vi "LinDaten speichern und laden.vi"(6 "Aktion":enum16{"speichern", "laden"}(ring), 8 "error in (no error)":errorcluster caption="Fehler (Eingang, kein Fehler)", 9 "test Polynom":bool, 10 "Analysator":T2, 11 "selected path":path caption="Ausgewählter Pfad") -> (0 "error out":errorcluster caption="Fehler (Ausgang)", 1 "Daten zum Speichern":string[](array[string]), 2 "LIN Protokoll Daten":T4 {"zusätzliche Zeitdauer Erster Punkt" format="%#_5g"; "Lin Modus" items=["Cal Gas to PNS", "Cal Gas to Samplepoint", "Measure"]; "Gas Ablaufdatum" format="%<%d.%m.%Y>T"; "HovaCAL Flow AutoLin"."HovaCAL Flow Input Cluster" format="%.2f"; "Gasflasche" items=["----"=10000, "IAG MG"=0, "IAG NH3 3000"=1, "IAG NH3 2000"=2, "IAG NH3 200"=3]; "Conditions:" items=["field", "laboratory"]; "Kalibrierauswahl" items=["Inaktiv", "Aktiv"]; "Anzahl Stufen" format="%#_5g"; "Zeitdauer Stufe" format="%#_5g"; "Verdünnungsgas" items=["N2", "O2"]; "Komponentenauswahl"."Konzentration" format="%#.6f"; "Gasnummer:" min=1 max=5; "Prüfgas Konzentration" format="%#.6f"; "Polynomkoeff." format="%#_18f"}, 3 "MessDaten Array":string[][][](array[string]), 4 "Ident Cluster":T18, 5 "Setup Daten-Cluster":T3, 7 "Settings Cluster":T1)   [LabVIEW 2020, in "Linearisierung v2.lvlib"]
uses:
  Linearisierung v2.lvlib
  SpanEinstellungen/LIN Loading Errors.ctl
  Lin-Polynom Daten.ctl
  KomponentenArray.ctl
  Visualisierungs Elemente/Auswahlfeld.ctl
  Visualisierungs Elemente/Zahlen-Eingabefeld.ctl
  EPA Optionsfeld.ctl
  Gasteiler/HovaCal/AutoLin Hovacal.ctl
  Kalibrieroption.ctl
  EPA1065-307/Condition.ctl
  Seiten/System Einstellungen V2/Konfig Gasflasche.ctl
  Seiten/System Einstellungen V2/Gasflasche Auswahl.ctl
  Gasteiler/HovaCAL_Interface/Controls/Flow Einstellung.ctl
  Gasteiler/HovaCAL_Interface/Controls/Pump state.ctl
  Seiten/CalGas Aufschaltung/Lin Modus.ctl
  SpanEinstellungen/LIN Loading Setup Data.ctl
  Seiten/System Einstellungen V2/Analysatoren.ctl
  Aktion Lin Daten aufarbeiten.ctl
  Seiten/FT-IR/FGV FT-IR Gasliste Aktionen.ctl
  Seiten/FT-IR/FGV FT-IR Aktionen.ctl
  Seiten/System Einstellungen V2/Aktioen FGV System Konstanten.ctl
  Seiten/System Einstellungen V2/Aktion FGV SystemEinstellungenV2.ctl
  Gasteiler/Aktionen FGV Gasteiler Daten.ctl
  PDF_Interface/PDF Protokoll Standard Kopf Gasflasche Auswahl.ctl
  SpanEinstellungen/Aktion FGV SpanEinstellungen.ctl
  Seiten/FT-IR/Span/Aktion FGV Span.ctl
  <vilib>/Utility/file.llb/Read Delimited Spreadsheet (string).vi
  Seiten/FT-IR/FT-IR.lvlib
  Seiten/System Einstellungen V2/System Einstellungen V2.lvlib
  Gasteiler/Gasteiler.lvlib
  PDF_Interface/PDF Interface.lvlib
  SpanEinstellungen/SpanEinstellungen.lvlib
  Seiten/FT-IR/Span/Spanfaktor.lvlib
  Protokoll/Protokoll.lvlib
  Gasteiler/HovaCal/HovaCal.lvlib
  EPA1065-307/Linearity verification 1065-307.lvlib
  Gasteiler/HovaCAL_Interface/Controls/Controls.lvlib
  Seiten/CalGas Aufschaltung/CalGas Aufschaltung.lvlib
panel:
  # "%"
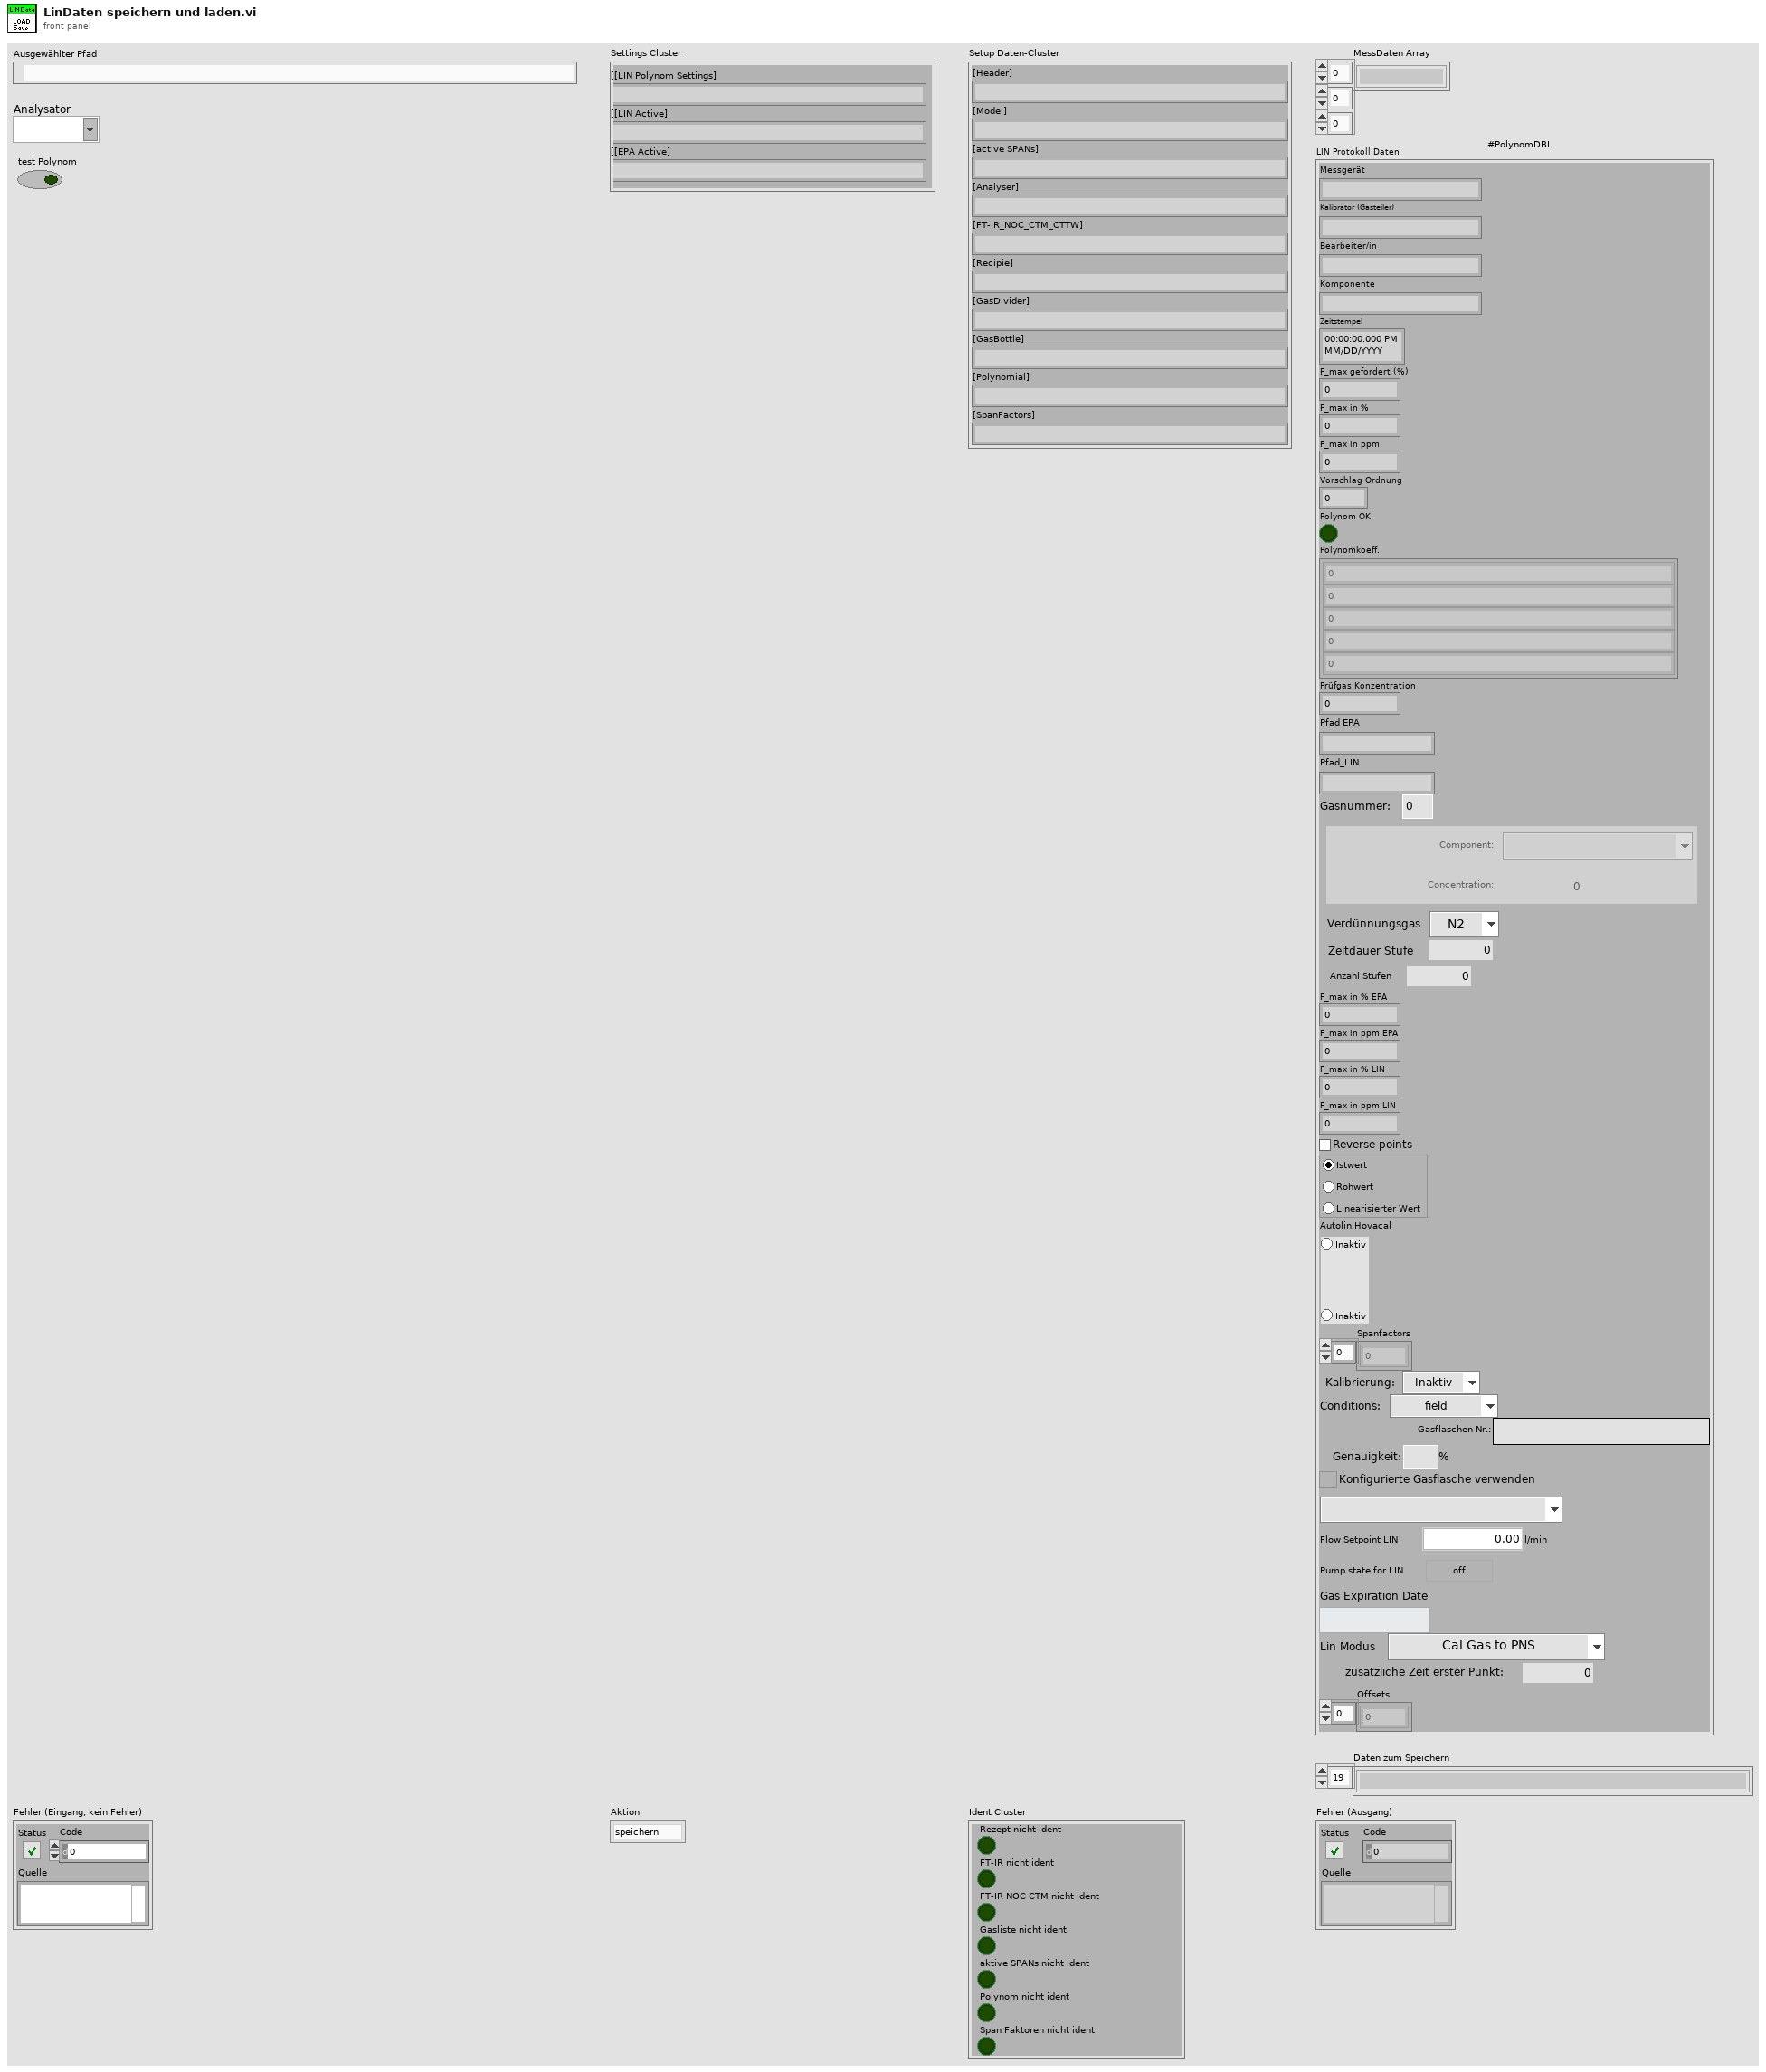
[diagram p1: front panel]
types:
  T1 = cluster{"[[LIN Polynom Settings]":string, "[[LIN Active]":string, "[[EPA Active]":string}
  T2 = typedef "System Einstellungen V2.lvlib/Analysatoren.ctl" = string
  T3 = typedef "Linearisierung v2.lvlib/SpanEinstellungen.lvlib/LIN Loading Setup Data.ctl" = cluster{"[Header]":string, "[Model]":string, "[active SPANs]":string, "[Analyser]":string, "[FT-IR_NOC_CTM_CTTW]":string, "[Recipie]":string, "[GasDivider]":string, "[GasBottle]":string, "[Polynomial]":string, "[SpanFactors]":string}
  T4 = typedef "Linearisierung v2.lvlib/Lin-Polynom Daten.ctl" = cluster{"Messgerät":string, "Kalibrator (Gasteiler)":string, "Bearbeiter/in":string, "Komponente":string, "Zeitstempel":timestamp, "F_max gefordert (%)":sgl, "F_max in %":sgl, "F_max in ppm":sgl, "Vorschlag Ordnung":i32, "Polynom OK":bool, "Polynomkoeff.":dbl[], "Prüfgas Konzentration":dbl, "Pfad EPA":string, "Pfad_LIN":string, "Gasnummer:":u8, "Komponentenauswahl":T5, "Verdünnungsgas":T7, "Zeitdauer Stufe":T8, "Anzahl Stufen":T8, "F_max in % EPA":sgl, "F_max in ppm EPA":sgl, "F_max in % LIN":sgl, "F_max in ppm LIN":sgl, "Punkte umkehren":bool, "EPA Optionsfeld":T9, "Autolin Hovacal":T10, "Spanfactors":sgl[], "Kalibrierauswahl":T11, "Conditions:":T12, "Gasflaschen Nr.:":string, "Bottle Accuracy":dbl, "Konfig Gasflasche":T13, "Gasflasche":T14, "HovaCAL Flow AutoLin":T15, "MFC Output":T16, "Gas Ablaufdatum":timestamp, "Lin Modus":T17, "zusätzliche Zeitdauer Erster Punkt":sgl, "Offsets":sgl[]}
  T5 = typedef "Linearisierung v2.lvlib/KomponentenArray.ctl" = cluster{"Komponente:":T6, "Konzentration":dbl}[]
  T6 = typedef "Auswahlfeld.ctl" = u16
  T7 = typedef "Linearisierung v2.lvlib/Gasteiler.lvlib/Prüfgas in.ctl" = u16
  T8 = typedef "Zahlen-Eingabefeld.ctl" = sgl
  T9 = typedef "Linearisierung v2.lvlib/EPA Optionsfeld.ctl" = enum32{"Istwert", "Rohwert", "Linearisierter Wert"}
  T10 = typedef "Linearisierung v2.lvlib/Gasteiler.lvlib/HovaCal.lvlib/AutoLin Hovacal.ctl" = enum32{"Keine Auswahl", "Optionsauswahl 1", "Optionsauswahl 2"}
  T11 = typedef "Linearisierung v2.lvlib/Kalibrieroption.ctl" = u16
  T12 = typedef "Linearisierung v2.lvlib/Linearity verification 1065-307.lvlib/Condition.ctl" = u16
  T13 = typedef "System Einstellungen V2.lvlib/Konfig Gasflasche.ctl" = bool
  T14 = typedef "System Einstellungen V2.lvlib/Gasflasche Auswahl.ctl" = u16
  T15 = typedef "Linearisierung v2.lvlib/Gasteiler.lvlib/HovaCAL_Interface.lvlib/Controls.lvlib/Flow Einstellung.ctl" = cluster{"HovaCAL Flow Input Cluster":dbl}
  T16 = typedef "Linearisierung v2.lvlib/Gasteiler.lvlib/HovaCAL_Interface.lvlib/Controls.lvlib/Pump state.ctl" = cluster{"Run":bool}
  T17 = typedef "CalGas Aufschaltung.lvlib/Lin Modus.ctl" = u16
  T18 = typedef "Linearisierung v2.lvlib/SpanEinstellungen.lvlib/LIN Loading Errors.ctl" = cluster{"Rezept nicht ident":bool, "FT-IR nicht ident":bool, "FT-IR NOC CTM nicht ident":bool, "Gasliste nicht ident":bool, "aktive SPANs nicht ident":bool, "Polynom nicht ident":bool, "Span Faktoren nicht ident":bool}
  T19 = typedef "Linearisierung v2.lvlib/Protokoll.lvlib/Aktion LIN Polynom Ordnung je Komponente für Protokoll.ctl" = enum16{"lesen", "schreiben", "init", "schreiben viewonly", "init initial"}
  T20 = typedef "Linearisierung v2.lvlib/SpanEinstellungen.lvlib/Aktion FGV SpanEinstellungen.ctl" = enum16{"lesen", "schreiben", "laden", "speichern", "RegisterRef", "automatisch", "init", "PDF Params", "Punkte umkehren"}
  T21 = typedef "PDF Interface.lvlib/PDF Protokoll Standard Kopf Gasflasche Auswahl.ctl" = cluster{"Gasflaschen Name":string, "Gasflaschen Nummer":string, "Gasnummer Index":i32}
  T22 = typedef "Linearisierung v2.lvlib/Gasteiler.lvlib/Aktionen FGV Gasteiler Daten.ctl" = enum16{"lesen", "Gasteiler Daten", "Seriellen Param.", "MB-Endwert", "laden", "speichern", "Anforderung", "TCP", "Aufzeichnung Start"}
  T23 = typedef "System Einstellungen V2.lvlib/Aktion FGV SystemEinstellungenV2.ctl" = enum16{"lesen", "Analysatoren schreiben", "Analysator ändern", "Analysatoren löschen", "laden", "speichern", "Untertitel", "Analysatoren", "Neue Analysatoren", "Gasteiler schreiben", "Gasteiler ändern", "Gasteiler löschen", "Gasteiler", "Gasteiler exportieren", "Gasteiler importieren"}
  T24 = typedef "System Einstellungen V2.lvlib/Aktioen FGV System Konstanten.ctl" = enum16{"lesen", "laden", "speichern", "Sprache"}
  T25 = typedef "FT-IR.lvlib/FGV FT-IR Aktionen.ctl" = enum16{"lesen", "NOG setzen", "NOS setzen", "Initialisieren", "speichern", "ALLES setzen", "FT-IR Spektrum loggen", "Komm Stoppen", "Spektrum LogKonfig"}
  T26 = typedef "FT-IR.lvlib/FGV FT-IR Gasliste Aktionen.ctl" = enum16{"lesen", "Gasliste FT-IR", "Gasliste ausgelesen", "laden", "speichern", "löschen"}
  T27 = typedef "Linearisierung v2.lvlib/Aktion Lin Daten aufarbeiten.ctl" = enum16{"lesen", "Protkolldaten", "speichern", "laden", "EPA auswerten", "Tabelle schreiben", "Lin auswerten", "Tab init", "Stufentabelle", "EPA aktiviert", "Nachbehandlung laden", "Tabelle löschen", "Istwerte löschen", "Zeile löschen", "Zeile einfügen", "LIN aktiviert", "LIN/EPA aktiv laden", "EGAK Tab", "LIN übernehmen", "Tab init ohne Stufen"}
  T28 = typedef "FT-IR.lvlib/Spanfaktor.lvlib/Aktion FGV Span.ctl" = enum16{"lesen", "Span", "Seite aktiv", "Offset", "FGV aktualisiert", "Aktualisierung aufheben"}
  T29 = typedef "System Einstellungen V2.lvlib/Gasteiler.ctl" = cluster{"Gasteiler Name":string, "Gasteiler Type":string, "Gasteiler Seriennummer":string, "Gasteiler Letzte Wartung":timestamp}
  T30 = cluster{"GasteilerDefinitionsListe":T29[], "GasteilerDefinitionTextliste":string[][], "Gasteiler Strings And Values":cluster{"String":string, "Wert":string}[]}
  T31 = typedef "Linearisierung v2.lvlib/Gasteiler.lvlib/Gasteiler Daten.ctl" = cluster{"Gasteiler":T32, "Gasteiler Stufen":T33, "Gasteiler Type":T34, "Konfig Gasteiler":T35, "Gasteiler Span Eingänge":u16}
  T32 = typedef "String - Eingabefeld.ctl" = string
  T33 = typedef "Linearisierung v2.lvlib/Gasteiler.lvlib/Gasteiler Stufen.ctl" = u16
  T34 = typedef "Linearisierung v2.lvlib/GasteilerType.ctl" = u16
  T35 = typedef "System Einstellungen V2.lvlib/Gasteiler Auswahl.ctl" = u16
  T36 = typedef "Linearisierung v2.lvlib/AktivArray.ctl" = T37[]
  T37 = typedef "Linearisierung v2.lvlib/AktivButton.ctl" = bool
  T38 = typedef "String - Ausgabefeld.ctl" = string
  T39 = cluster{"Modell":string, "ProjektNummer":string, "Software Version":string, "Seriennummer":string}
  T40 = typedef "Linearisierung v2.lvlib/SpanEinstellungen.lvlib/SpanInletCluster.ctl" = cluster{"Span Inlet Active":T13, "Analysator":T2, "Konfig Gasflasche":T13, "Gasflasche":T14, "Gasflaschen Nr.:":string, "Ablaufdatum":timestamp, "Komponenten":T41, "Zeitdauer Stufen":sgl, "Max Fehler":sgl, "Anzahl Stufen":sgl, "Trägergas":T44, "zusätzliche Zeitdauer Erster Punkt":sgl}
  T41 = typedef "Linearisierung v2.lvlib/SpanEinstellungen.lvlib/Komponentencluster mit Formel.ctl" = cluster{"Komponente 1":T42, "Komponente 2":T42, "Komponente 3":T42, "Komponente 4":T42, "Komponente 5":T42}
  T42 = typedef "Linearisierung v2.lvlib/SpanEinstellungen.lvlib/Komponentenauswahl mit Formel.ctl" = cluster{"Komponente:":u16, "Summenformel":T32, "Konzentration IST":dbl, "Einheit":T43, "Genauigkeit":dbl}
  T43 = typedef "Linearisierung v2.lvlib/SpanEinstellungen.lvlib/Einheit.ctl" = enum16{"ppm", "%"}
  T44 = typedef "System Einstellungen V2.lvlib/Traegergas.ctl" = string
  T45 = typedef "Linearisierung v2.lvlib/Auswahl Polynom Ordnung.ctl" = enum16{"autom.", "raw", "actual", "1", "2", "3", "4"}
  T46 = cluster{"active SPAN Idx":i32, "active Component Index":i32}
  T47 = cluster{"spreadsheet string":string, "spreadsheet string":string, "spreadsheet string":string, "spreadsheet string":string, "spreadsheet string":string, "spreadsheet string":string, "spreadsheet string":string, "spreadsheet string":string, "spreadsheet string":string, "spreadsheet string":string}
  T48 = cluster{"spreadsheet string":string, "spreadsheet string":string, "spreadsheet string":string}
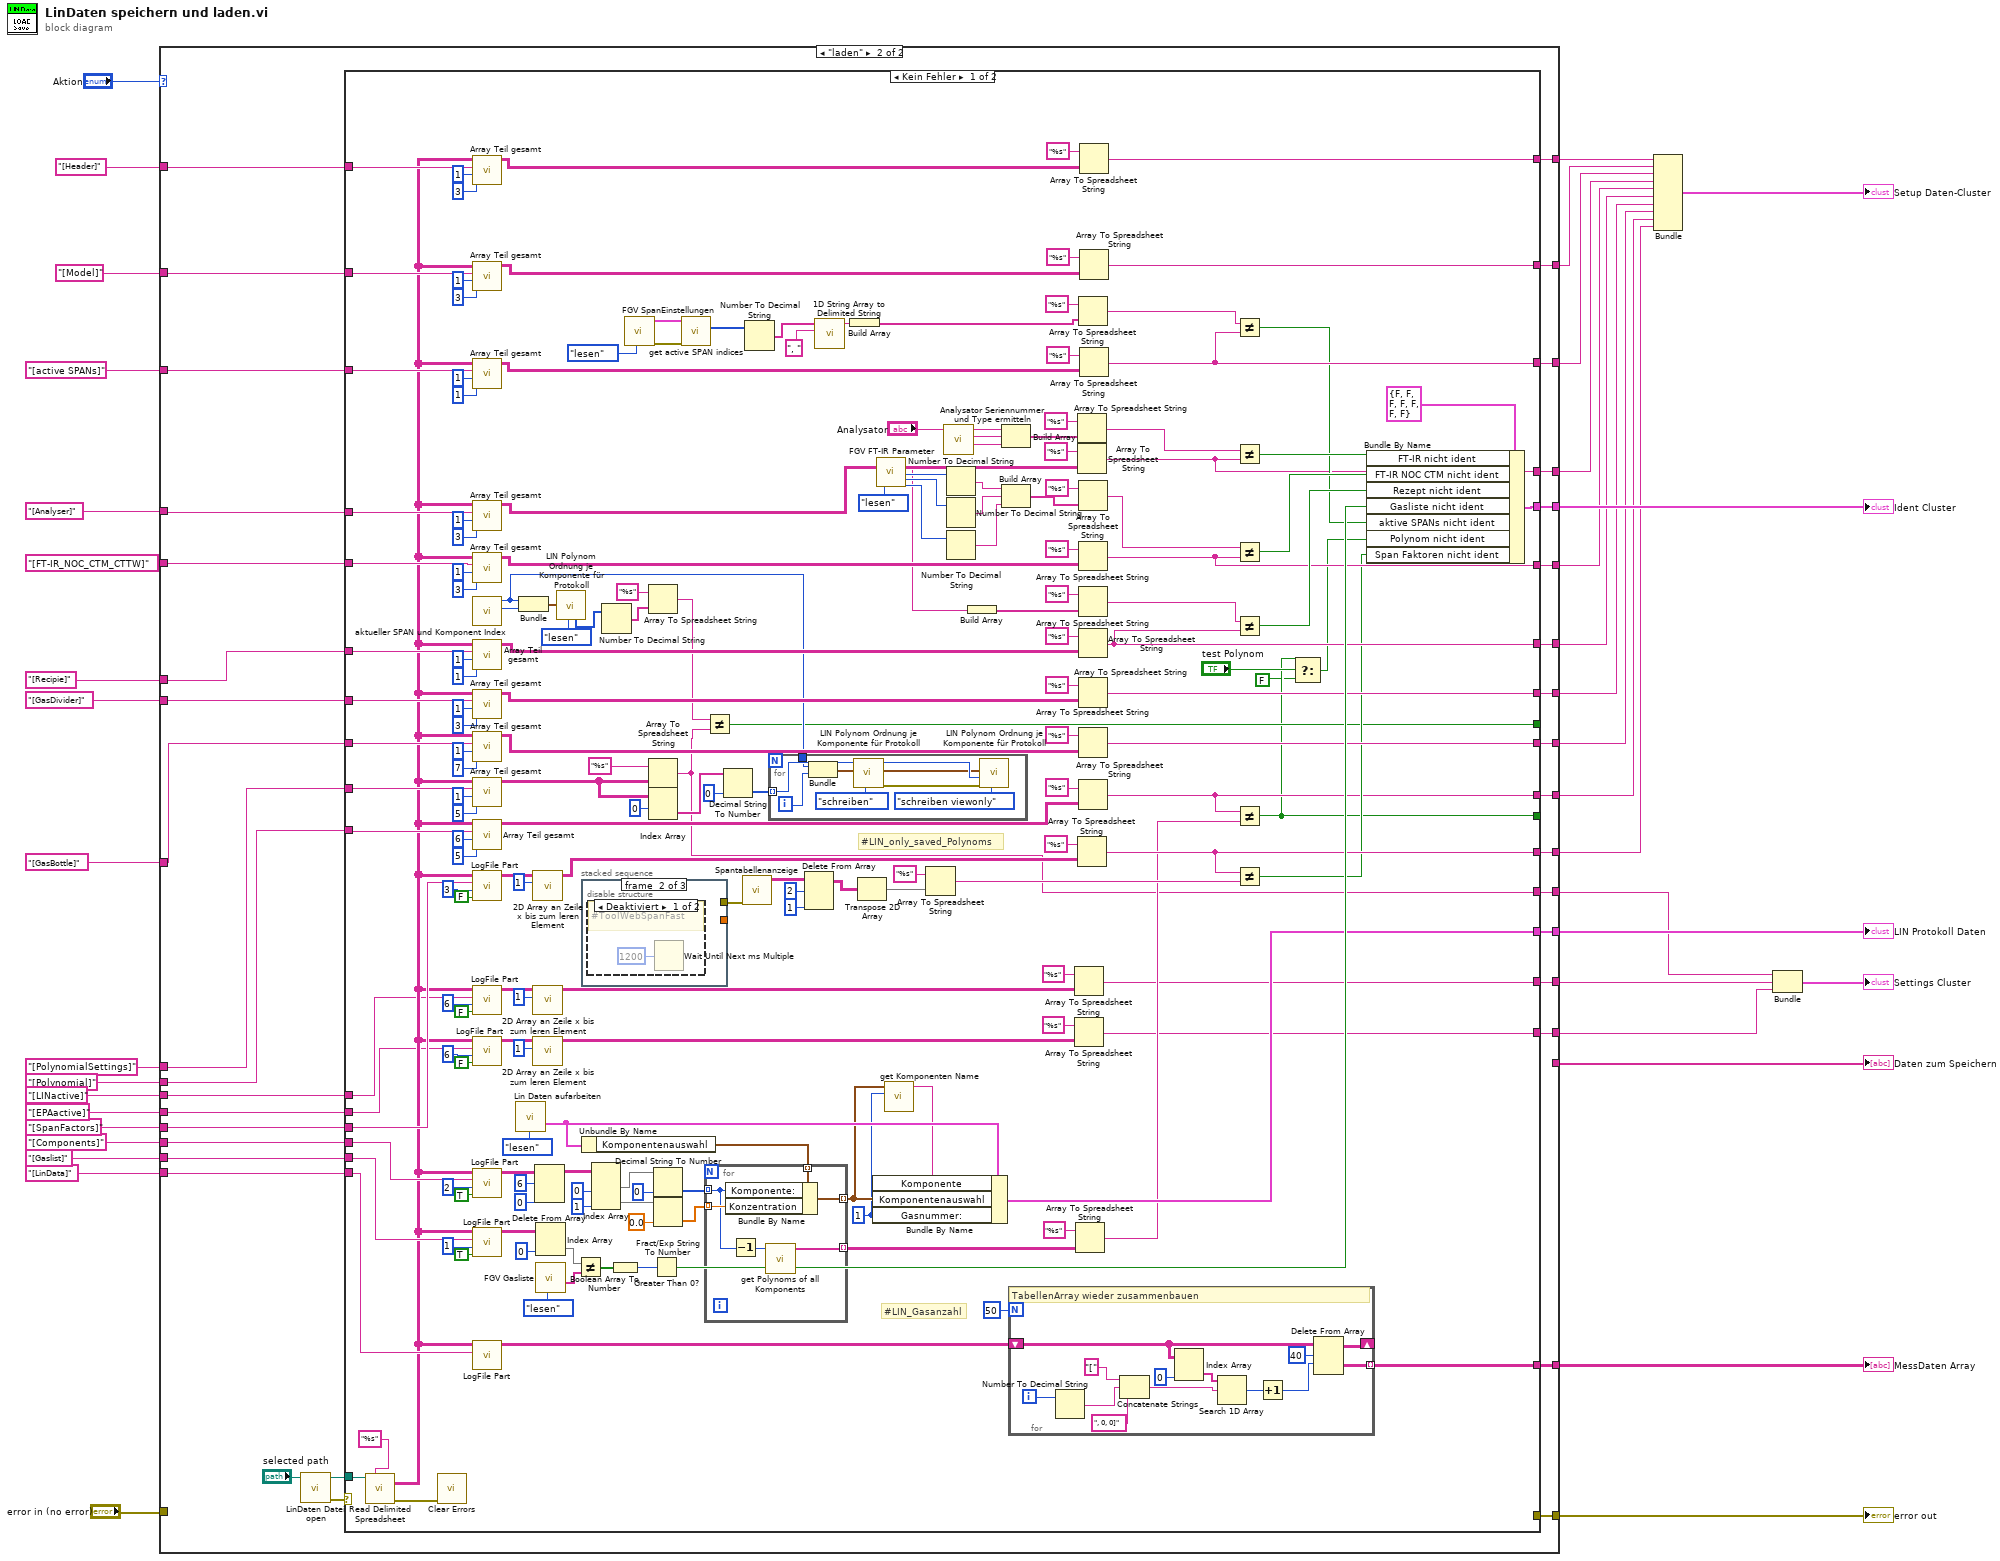
[diagram p0: block diagram]
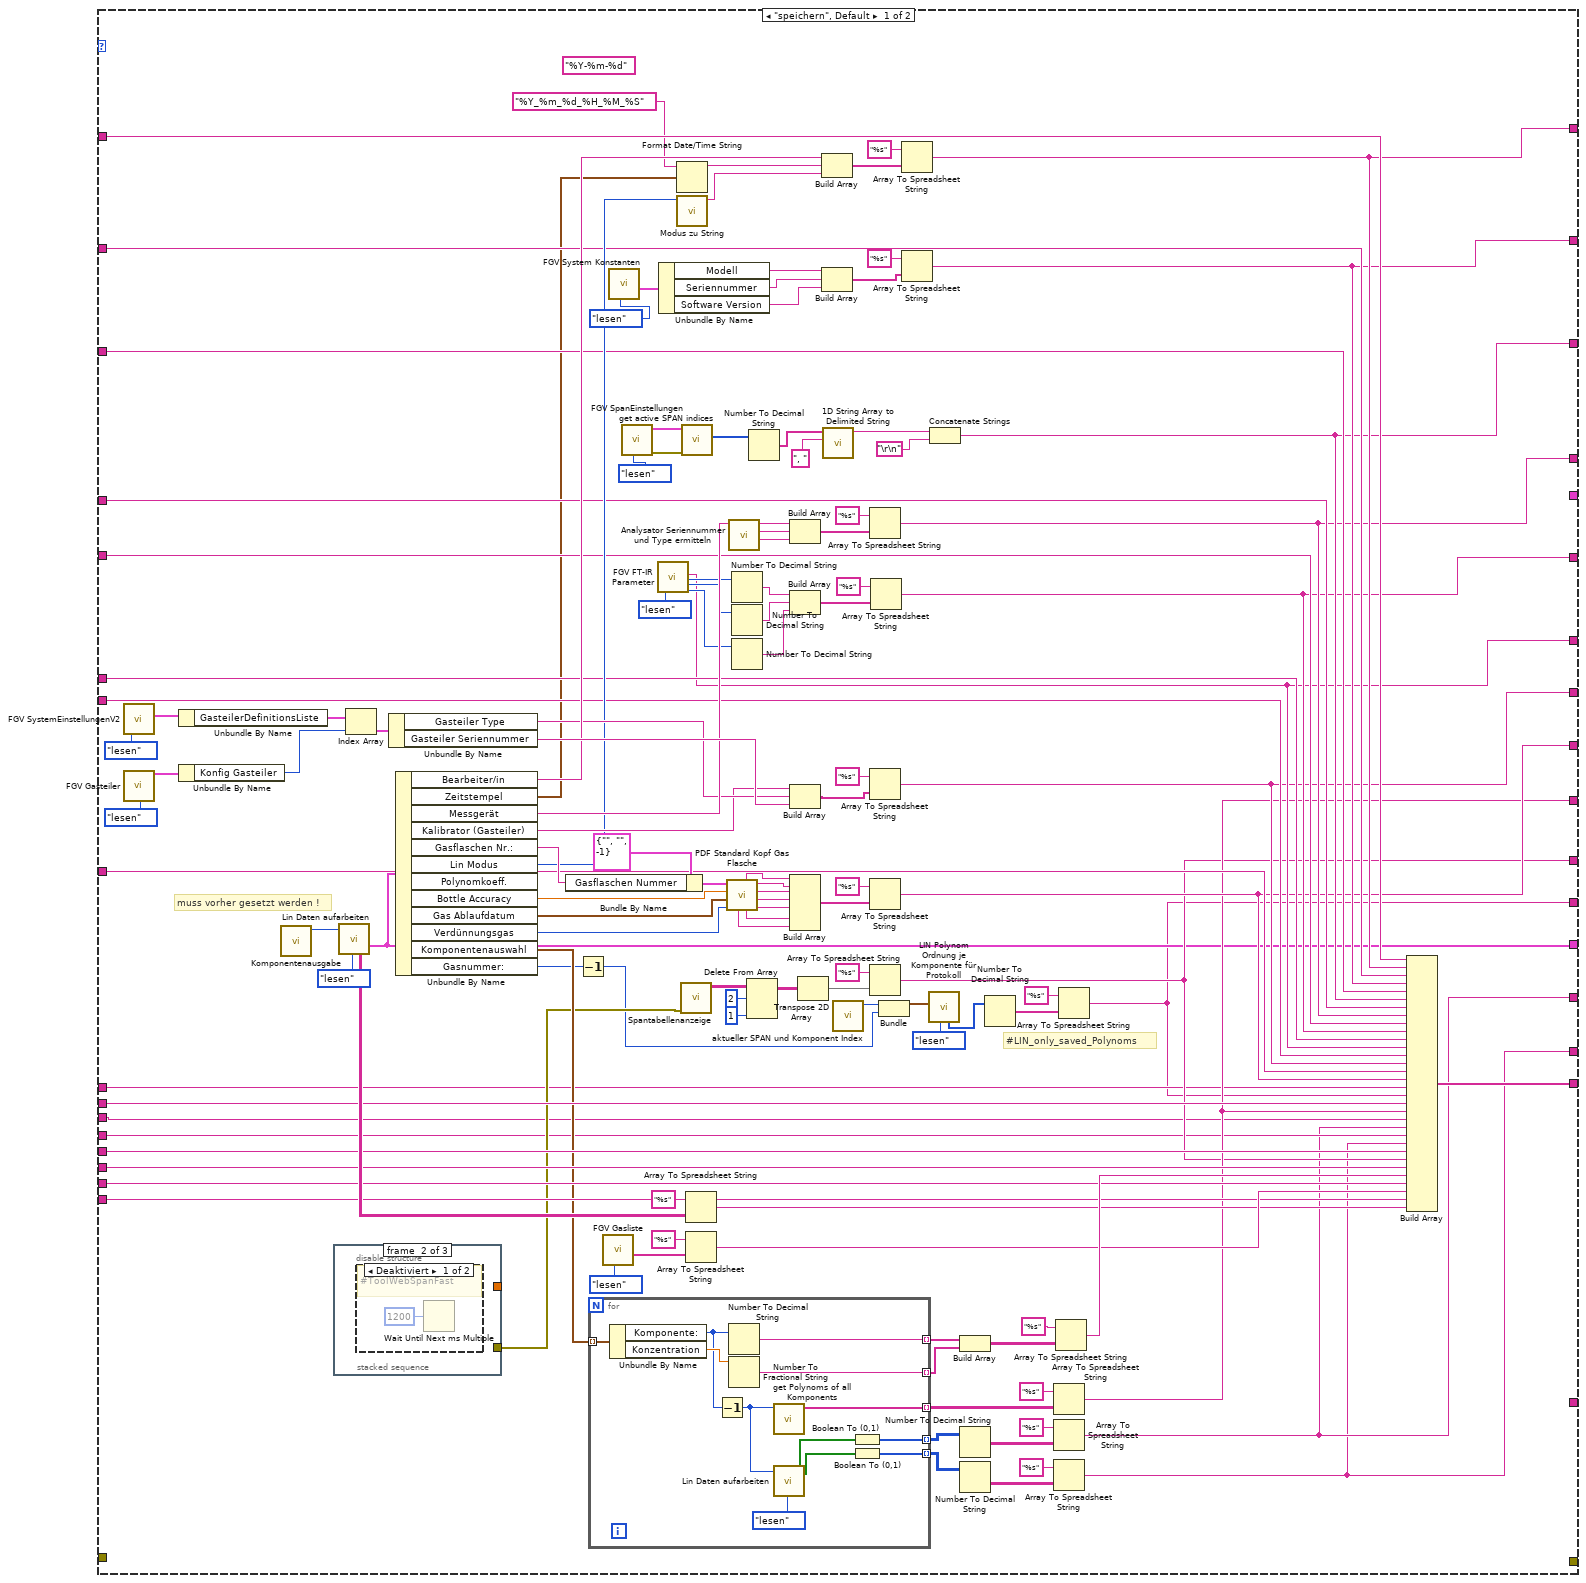
[diagram p2: hidden frame]
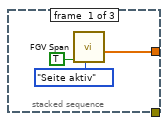
[diagram p3: hidden frame]
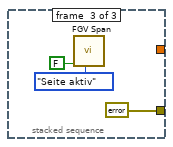
[diagram p5: hidden frame]
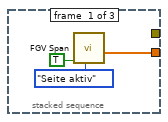
[diagram p6: hidden frame]
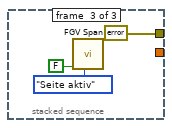
[diagram p8: hidden frame]
diagram:
  n1 = case shown="\"laden\"" "Aktion" {
    tunnel: [_ w225] -> w37
    tunnel: "[Header]" -> [w99 w213]
    tunnel: "[Model]" -> [w98 w214]
    tunnel: "[Analyser]" -> [w97 w215]
    tunnel: "[FT-IR_NOC_CTM_CTTW]" -> [w96 w216]
    tunnel: "[Recipie]" -> [w95 w217]
    tunnel: "[GasDivider]" -> [w94 w218]
    tunnel: "[GasBottle]" -> [w93 w219]
    tunnel: "[Polynomial]" -> [w92 w220]
    tunnel: "[SpanFactors]" -> [w91 w221]
    tunnel: "[Components]" -> [w90 w222]
    tunnel: "[Gaslist]" -> [w89 w224]
    tunnel: "[LinData]" -> [w88 w223]
    tunnel: [_ w212] -> w24
    tunnel: [w87 _] -> w23
    tunnel: "[active SPANs]" -> [w78 w210]
    tunnel: [w67 w209] -> w21
    tunnel: [_ w208] -> w20
    tunnel: [w77 w207] -> w19
    tunnel: [w76 w206] -> w18
    tunnel: [w75 w205] -> w17
    tunnel: [w71 w204] -> w13
    tunnel: [w70 w203] -> w12
    tunnel: [w69 w202] -> w11
    tunnel: [w68 w201] -> w10
    tunnel: [w74 w200] -> w16
    tunnel: [w73 w199] -> w15
    tunnel: [w72 w198] -> w14
    tunnel: "[PolynomialSettings]" -> [w58 w197]
    tunnel: "[LINactive]" -> [w43 w196]
    tunnel: "[EPAactive]" -> [w42 w195]
    tunnel: "error in (no error)" -> [_ _]
    tunnel: [w41 w194] -> w4
    tunnel: [w40 w193] -> w3
    tunnel: [w39 w192] -> w2
    frame "speichern", Default {
      (unwired) "%Y-%m-%d" ("Zeitformatierungs-String (%c)")
      # "muss vorher gesetzt werden !"
      # "#LIN_only_saved_Polynoms"
      n2 = call "FGV SystemEinstellungenV2.vi"("Aktion"=Aktion_FGV_SystemEinstellungenV2."lesen") -> ("Gasteiler"=w155:T30)  [unwired: 5 in, 5 out]
      n3 = call "FGV Gasteiler.vi"("Aktionen"=Aktionen_FGV_Gasteiler_Daten."lesen") -> ("Gasteiler Daten"=w153:T31)  [unwired: 11 in, 7 out]
      n4 = Unbundle By Name(w155) -> ("GasteilerDefinitionsListe"=w154:T29[])
      n5 = Unbundle By Name(w153) -> ("Konfig Gasteiler"=w151:T35)
      n6 = call "Komponentenausgabe.vi"() -> ("Gaskomponente"=w61:T6)  [unwired: 8 in, 3 out]
      n7 = stacked-sequence {
        tunnel: [w173 _ _] -> _
        tunnel: [_ _ errorcluster {"status"=FALSE, "code"=0, "source"=""} ("Fehlerkonstante")] -> w60
        frame #0 {
          n8 = call "FGV Span.vi"("Aktion"=Aktion_FGV_Span."Seite aktiv", "Aktiv"=TRUE) -> ("Offset"=w173:sgl[])  [unwired: 6 in, 3 out]
        }
        frame #1 {
          n9 = disable-structure shown="Deaktiviert" {
            frame Disabled {
              # "#ToolWebSpanFast"
              n10 = Wait Until Next ms Multiple(millisecond multiple=u32 1200 ("ms")) -> ()  [unwired: 1 out]
            }
            frame Enabled {
            }
          }
        }
        frame #2 {
          n11 = call "FGV Span.vi"("Aktion"=Aktion_FGV_Span."Seite aktiv", "Aktiv"=FALSE) -> ()  [unwired: 6 in, 4 out]
        }
      }
      n12 = call "Lin Daten aufarbeiten.vi"("Index (Seite)"=w61, "Aktionen"=Aktion_Lin_Daten_aufarbeiten."lesen") -> ("TabellenArray"=w171:string[][][], "Lin-Polynom"=w67:T4)  [unwired: 15 in, 9 out]
      n13 = Index Array(array=w154, index=w151) -> (element=w150:T29)
      n14 = Unbundle By Name(w150) -> ("Gasteiler Type"=w123:string, "Gasteiler Seriennummer"=w149:string)
      n15 = Unbundle By Name(w67) -> ("Bearbeiter/in"=w135:string, "Zeitstempel"=w63:timestamp, "Messgerät"=w133:string, "Kalibrator (Gasteiler)"=w122:string, "Gasflaschen Nr.:"=w143:string, "Lin Modus"=w101:T17, "Bottle Accuracy"=w103:dbl, "Gas Ablaufdatum"=w104:timestamp, "Verdünnungsgas"=w102:T7, "Komponentenauswahl"=w62:T5, "Gasnummer:"=w53:u8)  [unwired: 1 out]
      n16 = Bundle By Name(cluster=T21 {"Gasflaschen Name"="", "Gasflaschen Nummer"="", "Gasnummer Index"=-1} ("Gaschflasche Auswahl Cluster"), "Gasflaschen Nummer"=w143) -> (w147:T21)
      n17 = Decrement(x=w53) -> (x-1=w52:u8)
      n18 = for {
        tunnel: w62 -> [w191] mode=indexing
        tunnel: [w189] -> w164 mode=indexing
        tunnel: [w188] -> w165 mode=indexing
        tunnel: [w187] -> w50 mode=indexing
        tunnel: [w180] -> w48 mode=indexing
        tunnel: [w181] -> w49 mode=indexing
        n19 = Unbundle By Name(w191) -> ("Komponente:"=w185:T6, "Konzentration"=w190:dbl)
        n20 = Decrement(x=w185) -> (x-1=w184:T6)
        n21 = Number To Decimal String(number=w185) -> (decimal integer string=w188:string)  [unwired: 1 in]
        n22 = Number To Fractional String(number=w190) -> (F-format string=w189:string)  [unwired: 3 in]
        n23 = call "get Polynoms of all Komponents.vi"("Komponente"=w184) -> ("Polynom Array"=w187:string[])  [unwired: 10 in]
        n24 = call "Lin Daten aufarbeiten.vi"("Index (Seite)"=w184, "Aktionen"=Aktion_Lin_Daten_aufarbeiten."lesen") -> ("Aktiv EPA"=w183:T36, "Aktiv LIN"=w182:bool[])  [unwired: 15 in, 9 out]
        n25 = Boolean To (0,1)(Boolean=w182) -> (0, 1=w181:i16[])
        n26 = Boolean To (0,1)(Boolean=w183) -> (0, 1=w180:i16[])
      }
      n27 = call "FGV Gasliste.vi"("Aktionen"=FGV_FT-IR_Gasliste_Aktionen."lesen") -> ("Aktuelle Gasliste gesamt"=w167:T38[])  [unwired: 8 in, 2 out]
      n28 = call "FGV System Konstanten.vi"("Aktionen"=Aktioen_FGV_System_Konstanten."lesen") -> ("Cluster out"=w158:T39)  [unwired: 6 in, 4 out]
      n29 = call "FGV SpanEinstellungen.vi"("Aktion"=Aktion_FGV_SpanEinstellungen."lesen") -> ("error out"=w84:errorcluster, "SpanInletClusterArray out"=w85:T40[])  [unwired: 6 in, 3 out]
      n30 = call "FGV FT-IR Parameter.vi"("Aktion"=FGV_FT-IR_Aktionen."lesen") -> ("Current Recipe"=w72:string, "NoOfScan"=w129:u32, "Zykluszeit Messdatenverteiler"=w128:u32, "Zykluszeit ToolWeb"=w127:u32)  [unwired: 11 in, 4 out]
      n31 = Unbundle By Name(w158) -> ("Modell"=w142:string, "Seriennummer"=w141:string, "Software Version"=w140:string)
      n32 = Format Date/Time String(time format string (%c)="%Y_%m_%d_%H_%M_%S" ("Zeitformatierungs-String (%c)"), seconds (now)=w63) -> (date/time string=w134:string)  [unwired: 1 in]
      n33 = call "Modus zu String.vi"("Modus"=w101) -> ("Modus String"=w100:string)  [unwired: 10 in]
      n34 = call "Spantabellenanzeige.vi"("error in (no error)"=w60) -> ("SpanTabelle"=w146:T38[][])  [unwired: 9 in, 1 out]
      n35 = call "get active SPAN indices.vi"("error in (no error)"=w84, "SpanInletClusterArray in"=w85) -> ("Index active SPAN"=w83:i32[])  [unwired: 7 in, 2 out]
      n36 = Array To Spreadsheet String(array=w171, 3:"%s" ("Format-String")) -> (spreadsheet string=w160:string)  [unwired: 1 in]
      n37 = Array To Spreadsheet String(array=w167, 3:"%s" ("Format-String")) -> (spreadsheet string=w161:string)  [unwired: 1 in]
      n38 = call "PDF Standard Kopf Gas Flasche.vi"("Verdünnungsgas"=w102, "Ablaufdatum"=w104, "Genauigkeit in"=w103, "Gaschflasche Auswahl Cluster"=w147) -> ("Konzentration"=w111:string, "Ablaufdatum"=w112:string, "Genauigkeit"=w113:string, "Chargennummer"=w115:string, "Gasauswahl"=w110:string, "Gasname für die Auswahl"=w114:string, "Trägergas"=w109:T44)  [unwired: 1 in]
      n39 = call "Analysator Seriennummer und Type ermitteln.vi"("Analysator"=w133) -> ("Seriennummer"=w130:string, "Type"=w131:string, "Name für Protokoll"=w132:string)  [unwired: 8 in]
      n40 = Number To Decimal String(number=w129) -> (decimal integer string=w126:string)  [unwired: 1 in]
      n41 = Number To Decimal String(number=w128) -> (decimal integer string=w125:string)  [unwired: 1 in]
      n42 = Number To Decimal String(number=w127) -> (decimal integer string=w124:string)  [unwired: 1 in]
      n43 = Delete From Array(array=w146, length=2 ("Länge"), index (col)=1 ("Deaktivierter Index (Spalte)")) -> (array with subset deleted=w66:T38[][])  [unwired: 1 in, 1 out]
      n44 = Number To Decimal String(number=w83) -> (decimal integer string=w82:string[])  [unwired: 1 in]
      n45 = Build Array(w132, w131, w130) -> (w106:string[])
      n46 = Build Array(w126, w125, w124) -> (w120:string[])
      n47 = Build Array(w122, w123, w149) -> (w118:string[])
      n48 = Build Array(w114, w115, w113, w112, w111, w110, w109) -> (w117:T44[])
      n49 = Transpose 2D Array(2D array=w66) -> (transposed array=w65:T38[][])
      n50 = Build Array(w135, w134, w100) -> (w137:string[])
      n51 = Build Array(w142, w141, w140) -> (w138:string[])
      n52 = call <vilib>:"1D String Array to Delimited String.vi"("delimiter"=", ", "string array"=w82) -> ("delimited string"=w80:string)  [unwired: 9 in]
      n53 = call "aktueller SPAN und Komponent Index.vi"() -> ("akt SPAN out"=w55:i32)  [unwired: 7 in, 4 out]
      n54 = Array To Spreadsheet String(array=w106, 3:"%s" ("Format-String")) -> (spreadsheet string=w74:string)  [unwired: 1 in]
      n55 = Array To Spreadsheet String(array=w118, 3:"%s" ("Format-String")) -> (spreadsheet string=w71:string)  [unwired: 1 in]
      n56 = Array To Spreadsheet String(array=w117, 3:"%s" ("Format-String")) -> (spreadsheet string=w70:string)  [unwired: 1 in]
      n57 = Array To Spreadsheet String(array=w65, 3:"%s" ("Format-String")) -> (spreadsheet string=w68:string)  [unwired: 1 in]
      n58 = Array To Spreadsheet String(array=w120, 3:"%s" ("Format-String")) -> (spreadsheet string=w73:string)  [unwired: 1 in]
      n59 = Bundle("akt SPAN out"=w55, w52) -> (w54:cluster{"akt SPAN out":i32, u8})  [unwired: 1 in]
      n60 = Array To Spreadsheet String(array=w137, 3:"%s" ("Format-String")) -> (spreadsheet string=w77:string)  [unwired: 1 in]
      n61 = Array To Spreadsheet String(array=w138, 3:"%s" ("Format-String")) -> (spreadsheet string=w76:string)  [unwired: 1 in]
      n62 = call "LIN Polynom Ordnung je Komponente für Protokoll.vi"("Aktion"=Aktion_LIN_Polynom_Ordnung_je_Komponente_für_Protokoll."lesen", "Index in"=w54) -> ("Polynom Ordnungen SPAN"=w51:T45[])  [unwired: 3 in, 6 out]
      n63 = Concatenate Strings(w80, "\r\n") -> (w75:string)
      n64 = Build Array(w165, w164) -> (w163:string[][])
      n65 = Number To Decimal String(number=w49) -> (decimal integer string=w46:string[][])  [unwired: 1 in]
      n66 = Number To Decimal String(number=w48) -> (decimal integer string=w44:string[][])  [unwired: 1 in]
      n67 = Number To Decimal String(number=w51) -> (decimal integer string=w56:string[])  [unwired: 1 in]
      n68 = Array To Spreadsheet String(array=w50, 3:"%s" ("Format-String")) -> (spreadsheet string=w69:string)  [unwired: 1 in]
      n69 = Array To Spreadsheet String(array=w46, 3:"%s" ("Format-String")) -> (spreadsheet string=w40:string)  [unwired: 1 in]
      n70 = Array To Spreadsheet String(array=w44, 3:"%s" ("Format-String")) -> (spreadsheet string=w39:string)  [unwired: 1 in]
      n71 = Array To Spreadsheet String(array=w163, 3:"%s" ("Format-String")) -> (spreadsheet string=w162:string)  [unwired: 1 in]
      n72 = Array To Spreadsheet String(array=w56, 3:"%s" ("Format-String")) -> (spreadsheet string=w41:string)  [unwired: 1 in]
      n73 = Build Array(w99, w77, w98, w76, w78, w75, w97, w74, w96, w73, w95, w72, w94, w71, w93, w70, w58, w41, w92, w69, w43, w40, w42, w39, w91, w68, w90, w162, w89, w161, w88, w160) -> (w87:string[])
    }
    frame "laden" {
      n74 = call "LinDaten Datei open.vi"("selected path (Eingang)"="selected path") -> ("Fehler (Ausgang)"=w226:errorcluster, "selected path (Ausgang)"=w227:path)  [unwired: 9 in]
      n75 = case shown="Kein Fehler" w226 {
        selector: w226 -> [_ w454]
        tunnel: w227 -> [w418 _]
        tunnel: [_ w454] -> w225
        tunnel: w224 -> [w333 _]
        tunnel: w223 -> [w330 _]
        tunnel: w222 -> [w339 _]
        tunnel: w221 -> [w278 _]
        tunnel: w220 -> [w342 _]
        tunnel: w219 -> [w347 _]
        tunnel: w218 -> [w354 _]
        tunnel: w217 -> [w358 _]
        tunnel: w216 -> [w361 _]
        tunnel: w215 -> [w364 _]
        tunnel: w214 -> [w365 _]
        tunnel: w213 -> [w368 _]
        tunnel: [w306 _] -> w201
        tunnel: [w373 _] -> w212
        tunnel: [w351 _] -> w207
        tunnel: [w350 _] -> w204
        tunnel: [w345 _] -> w203
        tunnel: [w303 _] -> w202
        tunnel: [w328 _] -> w206
        tunnel: w210 -> [w324 _]
        tunnel: [w318 _] -> w205
        tunnel: [w315 _] -> w209
        tunnel: [w314 _] -> w208
        tunnel: [w313 _] -> w200
        tunnel: [w312 _] -> w199
        tunnel: [w311 _] -> w198
        tunnel: w197 -> [w268 _]
        tunnel: [w257 _] -> _
        tunnel: [w231 _] -> _
        tunnel: w196 -> [w251 _]
        tunnel: w195 -> [w250 _]
        tunnel: [w242 _] -> w194
        tunnel: [w239 _] -> w193
        tunnel: [w236 _] -> w192
        frame No Error {
          w234 = u8 1 ("Gasnummer:")
          # "#LIN_only_saved_Polynoms"
          # "#LIN_Gasanzahl"
          n76 = call-poly <vilib>:"Read Delimited Spreadsheet.vi"("file path (dialog if empty)"=w418, "format (%s)"="%s" ("Format-String")) -> ("all rows"=w252:string[][], "error out"=w228:errorcluster)  [unwired: 8 in, 4 out]
          n77 = call <vilib>:"Clear Errors.vi"("error in (no error)"=w228) -> ()  [unwired: 5 in, 2 out]
          n78 = call "Array Teil gesamt.vi"("Spalten"=3, "Zeilen"=1, "Key"=w368, "Data"=w252) -> ("Teil Array (Ausgang)"=w298:string[][])  [unwired: 6 in, 1 out]
          n79 = call "Array Teil gesamt.vi"("Spalten"=3, "Zeilen"=1, "Key"=w365, "Data"=w252) -> ("Teil Array (Ausgang)"=w297:string[][])  [unwired: 6 in, 1 out]
          n80 = call "Array Teil gesamt.vi"("Spalten"=1, "Zeilen"=1, "Key"=w324, "Data"=w252) -> ("Teil Array (Ausgang)"=w296:string[][])  [unwired: 6 in, 1 out]
          n81 = call "Array Teil gesamt.vi"("Spalten"=3, "Zeilen"=1, "Key"=w364, "Data"=w252) -> ("Teil Array (Ausgang)"=w295:string[][])  [unwired: 6 in, 1 out]
          n82 = call "Array Teil gesamt.vi"("Spalten"=3, "Zeilen"=1, "Key"=w361, "Data"=w252) -> ("Teil Array (Ausgang)"=w294:string[][])  [unwired: 6 in, 1 out]
          n83 = call "aktueller SPAN und Komponent Index.vi"() -> ("akt Comp out"=w260:i32, "akt SPAN out"=w258:i32)  [unwired: 7 in, 3 out]
          n84 = call "Array Teil gesamt.vi"("Spalten"=1, "Zeilen"=1, "Key"=w358, "Data"=w252) -> ("Teil Array (Ausgang)"=w293:string[][])  [unwired: 6 in, 1 out]
          n85 = call "Array Teil gesamt.vi"("Spalten"=3, "Zeilen"=1, "Key"=w354, "Data"=w252) -> ("Teil Array (Ausgang)"=w292:string[][])  [unwired: 6 in, 1 out]
          n86 = call "Array Teil gesamt.vi"("Spalten"=7, "Zeilen"=1, "Key"=w347, "Data"=w252) -> ("Teil Array (Ausgang)"=w291:string[][])  [unwired: 6 in, 1 out]
          n87 = call "Array Teil gesamt.vi"("Spalten"=5, "Zeilen"=1, "Key"=w268, "Data"=w252) -> ("Teil Array (Ausgang)"=w264:string[][])  [unwired: 6 in, 1 out]
          n88 = call "Array Teil gesamt.vi"("Spalten"=5, "Zeilen"=6, "Key"=w342, "Data"=w252) -> ("Teil Array (Ausgang)"=w290:string[][])  [unwired: 6 in, 1 out]
          n89 = call "LogFile Part.vi"("as Column"=FALSE, "Länge"=3, "Key"=w278, "Data"=w252) -> ("Part Array"=w277:string[][])  [unwired: 7 in]
          n90 = call "LogFile Part.vi"("as Column"=FALSE, "Länge"=6, "Key"=w251, "Data"=w252) -> ("Part Array"=w248:string[][])  [unwired: 7 in]
          n91 = call "LogFile Part.vi"("as Column"=FALSE, "Länge"=6, "Key"=w250, "Data"=w252) -> ("Part Array"=w246:string[][])  [unwired: 7 in]
          n92 = call "LogFile Part.vi"("as Column"=TRUE, "Länge"=2, "Key"=w339, "Data"=w252) -> ("Part Array"=w336:string[][])  [unwired: 7 in]
          n93 = call "LogFile Part.vi"("as Column"=TRUE, "Länge"=1, "Key"=w333, "Data"=w252) -> ("Part Array"=w332:string[][])  [unwired: 7 in]
          n94 = call "LogFile Part.vi"("Key"=w330, "Data"=w252) -> ("Part Array"=w331:string[][])  [unwired: 9 in]
          n95 = call "Lin Daten aufarbeiten.vi"("Aktionen"=Aktion_Lin_Daten_aufarbeiten."lesen") -> ("Lin-Polynom"=w399:T4)  [unwired: 16 in, 10 out]
          n96 = Bundle("akt SPAN out"=w258, "akt Comp out"=w260) -> (w259:cluster{"akt SPAN out":i32, "akt Comp out":i32})  [unwired: 1 in]
          n97 = call "2D Array an Zeile x bis zum leren Element.vi"("Index (Zeile)"=1, "Part Array"=w277) -> ("Array gestutzt"=w276:string[][])  [unwired: 9 in]
          n98 = call "2D Array an Zeile x bis zum leren Element.vi"("Index (Zeile)"=1, "Part Array"=w248) -> ("Array gestutzt"=w240:string[][])  [unwired: 9 in]
          n99 = call "2D Array an Zeile x bis zum leren Element.vi"("Index (Zeile)"=1, "Part Array"=w246) -> ("Array gestutzt"=w237:string[][])  [unwired: 9 in]
          n100 = Delete From Array(array=w336, length=6 ("Länge"), index (row)=0 ("Index (Zeile)")) -> (deleted portion=w410:string[][])  [unwired: 1 in, 1 out]
          n101 = Index Array(array=w332, index (col)=0 ("Deaktivierter Index (Spalte)")) -> (element=w405:string[])  [unwired: 1 in]
          n102 = call "FGV Gasliste.vi"("Aktionen"=FGV_FT-IR_Gasliste_Aktionen."lesen") -> ("Aktuelle Gasliste gesamt"=w404:T38[])  [unwired: 8 in, 2 out]
          n103 = call "LIN Polynom Ordnung je Komponente für Protokoll.vi"("Aktion"=Aktion_LIN_Polynom_Ordnung_je_Komponente_für_Protokoll."lesen", "Index in"=w259) -> ("Polynom Ordnungen SPAN"=w244:T45[])  [unwired: 3 in, 6 out]
          n104 = Not Equal?(x=w405, y=w404) -> (x != y?=w403:bool[])
          n105 = stacked-sequence {
            tunnel: [w428 _ _] -> _
            tunnel: [_ _ errorcluster {"status"=FALSE, "code"=0, "source"=""} ("Fehlerkonstante")] -> w274
            frame #0 {
              n106 = call "FGV Span.vi"("Aktion"=Aktion_FGV_Span."Seite aktiv", "Aktiv"=TRUE) -> ("Offset"=w428:sgl[])  [unwired: 6 in, 3 out]
            }
            frame #1 {
              n107 = disable-structure shown="Deaktiviert" {
                frame Disabled {
                  # "#ToolWebSpanFast"
                  n108 = Wait Until Next ms Multiple(millisecond multiple=u32 1200 ("ms")) -> ()  [unwired: 1 out]
                }
                frame Enabled {
                }
              }
            }
            frame #2 {
              n109 = call "FGV Span.vi"("Aktion"=Aktion_FGV_Span."Seite aktiv", "Aktiv"=FALSE) -> ()  [unwired: 6 in, 4 out]
            }
          }
          n110 = Unbundle By Name(w399) -> ("Komponentenauswahl"=w398:T5)
          n111 = Index Array(array=w410, index (col) #1=0 ("Deaktivierter Index (Spalte)"), index (col) #2=1 ("Index (Spalte)")) -> (element #1=w411:string[], element #2=w412:string[])  [unwired: 2 in]
          n112 = Number To Decimal String(number=w244) -> (decimal integer string=w243:string[])  [unwired: 1 in]
          n113 = Boolean Array To Number(Boolean array=w403) -> (number=w402:u32)
          n114 = call "FGV SpanEinstellungen.vi"("Aktion"=Aktion_FGV_SpanEinstellungen."lesen") -> ("error out"=w322:errorcluster, "SpanInletClusterArray out"=w323:T40[])  [unwired: 6 in, 3 out]
          n115 = Array To Spreadsheet String(array=w243, 3:"%s" ("Format-String")) -> (spreadsheet string=w265:string)  [unwired: 1 in]
          n116 = Array To Spreadsheet String(array=w264, 3:"%s" ("Format-String")) -> (spreadsheet string=w242:string)  [unwired: 1 in]
          n117 = Index Array(array=w264, index (row)=0 ("Deaktivierter Index (Spalte)")) -> (element=w263:string[])  [unwired: 1 in]
          n118 = Greater Than 0?(x=w402) -> (x > 0?=w374:bool)
          n119 = Decimal String To Number(string=w411, default (0L)=u16 0 ("Standard (0 I32)")) -> (number=w397:u16[])  [unwired: 1 in, 1 out]
          n120 = Fract/Exp String To Number(string=w412, default (0 dbl)=sgl 0.0 ("Standard (0 DBL)")) -> (number=w396:sgl[])  [unwired: 2 in, 1 out]
          n121 = call "get active SPAN indices.vi"("error in (no error)"=w322, "SpanInletClusterArray in"=w323) -> ("Index active SPAN"=w321:i32[])  [unwired: 7 in, 2 out]
          n122 = for {
            tunnel: w398 -> [w440] mode=indexing
            tunnel: w397 -> [w437] mode=indexing
            tunnel: w396 -> [w439] mode=indexing
            tunnel: [w438] -> w235 mode=indexing
            tunnel: [w435] -> w245 mode=indexing
            n123 = Bundle By Name(cluster=w440, "Komponente:"=w437, "Konzentration"=w439) -> (w438:cluster{"Komponente:":T6, "Konzentration":dbl})
            n124 = Decrement(x=w437) -> (x-1=w436:u16)
            n125 = call "get Polynoms of all Komponents.vi"("Komponente"=w436) -> ("Polynom Array"=w435:string[])  [unwired: 10 in]
          }
          n126 = Not Equal?(x=w265, y=w242) -> (x != y?=w257:bool)
          n127 = Decimal String To Number(string=w263, default (0L)=u16 0 ("Standard (0 I32)")) -> (number=w261:u16[])  [unwired: 1 in, 1 out]
          n128 = call "Spantabellenanzeige.vi"("error in (no error)"=w274) -> ("SpanTabelle"=w310:T38[][])  [unwired: 9 in, 1 out]
          n129 = Number To Decimal String(number=w321) -> (decimal integer string=w320:string[])  [unwired: 1 in]
          n130 = for {
            tunnel: w261 -> [w425] mode=indexing
            tunnel: w258 -> [w419]
            i -> [w423]
            n131 = Bundle("akt SPAN out"=w419, w423) -> (w420:cluster{"akt SPAN out":i32, i32})  [unwired: 1 in]
            n132 = call "LIN Polynom Ordnung je Komponente für Protokoll.vi"("Aktion"=Aktion_LIN_Polynom_Ordnung_je_Komponente_für_Protokoll."schreiben", "Index in"=w420, "Polynom-Ordnung"=w425) -> ("error out"=w421:errorcluster, "Index out"=w422:T46, "Polynom-Ordnung out"=w424:T45)  [unwired: 2 in, 4 out]
            n133 = call "LIN Polynom Ordnung je Komponente für Protokoll.vi"("Aktion"=Aktion_LIN_Polynom_Ordnung_je_Komponente_für_Protokoll."schreiben viewonly", "error in (no error)"=w421, "Polynom-Ordnung view only"=w424, "Index in"=w422) -> ()  [unwired: 1 in, 7 out]
          }
          n134 = Delete From Array(array=w310, length=2 ("Länge"), index (col)=1 ("Deaktivierter Index (Spalte)")) -> (array with subset deleted=w300:T38[][])  [unwired: 1 in, 1 out]
          n135 = call <vilib>:"1D String Array to Delimited String.vi"("delimiter"=", ", "string array"=w320) -> ("delimited string"=w288:string)  [unwired: 9 in]
          n136 = Build Array(w288) -> (w287:string[])
          n137 = Transpose 2D Array(2D array=w300) -> (transposed array=w299:T38[][])
          n138 = call "FGV FT-IR Parameter.vi"("Aktion"=FGV_FT-IR_Aktionen."lesen") -> ("Current Recipe"=w283:string, "NoOfScan"=w391:u32, "Zykluszeit Messdatenverteiler"=w390:u32, "Zykluszeit ToolWeb"=w389:u32)  [unwired: 11 in, 4 out]
          n139 = call "get Komponenten Name.vi"("Gasnummer:"=w234, "Array"=w235) -> ("String - Ausgabefeld"=w233:T38)  [unwired: 9 in]
          n140 = Bundle By Name(cluster=w399, "Komponente"=w233, "Komponentenauswahl"=w235, "Gasnummer:"=w234) -> (w315:T4)
          n141 = Array To Spreadsheet String(array=w299, 3:"%s" ("Format-String")) -> (spreadsheet string=w305:string)  [unwired: 1 in]
          n142 = call "Analysator Seriennummer und Type ermitteln.vi"("Analysator"="Analysator") -> ("Seriennummer"=w392:string, "Type"=w393:string, "Name für Protokoll"=w394:string)  [unwired: 8 in]
          n143 = Number To Decimal String(number=w391) -> (decimal integer string=w388:string)  [unwired: 1 in]
          n144 = Number To Decimal String(number=w390) -> (decimal integer string=w387:string)  [unwired: 1 in]
          n145 = Number To Decimal String(number=w389) -> (decimal integer string=w386:string)  [unwired: 1 in]
          n146 = Build Array(w283) -> (w282:string[])
          n147 = Build Array(w394, w393, w392) -> (w382:string[])
          n148 = Build Array(w388, w387, w386) -> (w384:string[])
          n149 = for {
            N: 50 -> [_]
            shift-right: [w445] -> _
            shift-left: w331 -> [w449]
            tunnel: [w442] -> w314 mode=indexing
            i -> [w453]
            # "TabellenArray wieder zusammenbauen"
            n150 = Number To Decimal String(number=w453) -> (decimal integer string=w451:string)  [unwired: 1 in]
            n151 = Concatenate Strings("[", w451, ", 0, 0]") -> (w447:string)
            n152 = Index Array(array=w449, index (col)=0 ("Deaktivierter Index (Spalte)")) -> (element=w448:string[])  [unwired: 1 in]
            n153 = Search 1D Array(1D array=w448, element=w447) -> (index of element=w444:i32)  [unwired: 1 in]
            n154 = Increment(x=w444) -> (x+1=w443:i32)
            n155 = Delete From Array(array=w449, length=40 ("Länge"), index (row)=w443) -> (deleted portion=w442:string[][], array with subset deleted=w445:string[][])  [unwired: 1 in]
          }
          n156 = Array To Spreadsheet String(array=w240, 3:"%s" ("Format-String")) -> (spreadsheet string=w239:string)  [unwired: 1 in]
          n157 = Array To Spreadsheet String(array=w237, 3:"%s" ("Format-String")) -> (spreadsheet string=w236:string)  [unwired: 1 in]
          n158 = Array To Spreadsheet String(array=w245, 3:"%s" ("Format-String")) -> (spreadsheet string=w301:string)  [unwired: 1 in]
          n159 = Array To Spreadsheet String(array=w382, 3:"%s" ("Format-String")) -> (spreadsheet string=w381:string)  [unwired: 1 in]
          n160 = Array To Spreadsheet String(array=w295, 3:"%s" ("Format-String")) -> (spreadsheet string=w313:string)  [unwired: 1 in]
          n161 = Array To Spreadsheet String(array=w276, 3:"%s" ("Format-String")) -> (spreadsheet string=w306:string)  [unwired: 1 in]
          n162 = Array To Spreadsheet String(array=w287, 3:"%s" ("Format-String")) -> (spreadsheet string=w286:string)  [unwired: 1 in]
          n163 = Array To Spreadsheet String(array=w384, 3:"%s" ("Format-String")) -> (spreadsheet string=w380:string)  [unwired: 1 in]
          n164 = Array To Spreadsheet String(array=w294, 3:"%s" ("Format-String")) -> (spreadsheet string=w312:string)  [unwired: 1 in]
          n165 = Array To Spreadsheet String(array=w282, 3:"%s" ("Format-String")) -> (spreadsheet string=w284:string)  [unwired: 1 in]
          n166 = Array To Spreadsheet String(array=w293, 3:"%s" ("Format-String")) -> (spreadsheet string=w311:string)  [unwired: 1 in]
          n167 = Array To Spreadsheet String(array=w292, 3:"%s" ("Format-String")) -> (spreadsheet string=w350:string)  [unwired: 1 in]
          n168 = Array To Spreadsheet String(array=w291, 3:"%s" ("Format-String")) -> (spreadsheet string=w345:string)  [unwired: 1 in]
          n169 = Array To Spreadsheet String(array=w290, 3:"%s" ("Format-String")) -> (spreadsheet string=w303:string)  [unwired: 1 in]
          n170 = Array To Spreadsheet String(array=w298, 3:"%s" ("Format-String")) -> (spreadsheet string=w351:string)  [unwired: 1 in]
          n171 = Array To Spreadsheet String(array=w297, 3:"%s" ("Format-String")) -> (spreadsheet string=w328:string)  [unwired: 1 in]
          n172 = Array To Spreadsheet String(array=w296, 3:"%s" ("Format-String")) -> (spreadsheet string=w318:string)  [unwired: 1 in]
          n173 = Not Equal?(x=w286, y=w318) -> (x != y?=w317:bool)
          n174 = Not Equal?(x=w381, y=w313) -> (x != y?=w377:bool)
          n175 = Not Equal?(x=w380, y=w312) -> (x != y?=w376:bool)
          n176 = Not Equal?(x=w284, y=w311) -> (x != y?=w375:bool)
          n177 = Not Equal?(x=w303, y=w301) -> (x != y?=w231:bool)
          n178 = Not Equal?(x=w306, y=w305) -> (x != y?=w304:bool)
          n179 = Select(t=w231, s="test Polynom", f=FALSE ("Polynom nicht ident")) -> (s? t:f=w229:bool)
          n180 = Bundle By Name(cluster=T18 {"Rezept nicht ident"=FALSE, "FT-IR nicht ident"=FALSE, "FT-IR NOC CTM nicht ident"=FALSE, "Gasliste nicht ident"=FALSE, "aktive SPANs nicht ident"=FALSE, "Polynom nicht ident"=FALSE, "Span Faktoren nicht ident"=FALSE} ("Ident Cluster"), "FT-IR nicht ident"=w377, "FT-IR NOC CTM nicht ident"=w376, "Rezept nicht ident"=w375, "Gasliste nicht ident"=w374, "aktive SPANs nicht ident"=w317, "Polynom nicht ident"=w229, "Span Faktoren nicht ident"=w304) -> (w373:T18)
        }
        frame Error {
        }
      }
    }
  }
  "error out" <- w37
  "Ident Cluster" <- w24
  "Daten zum Speichern" <- w23
  "LIN Protokoll Daten" <- w21
  "MessDaten Array" <- w20
  n181 = Bundle("spreadsheet string"=w19, "spreadsheet string"=w18, "spreadsheet string"=w17, "spreadsheet string"=w16, "spreadsheet string"=w15, "spreadsheet string"=w14, "spreadsheet string"=w13, "spreadsheet string"=w12, "spreadsheet string"=w11, "spreadsheet string"=w10) -> (→"Setup Daten-Cluster":T47)  [unwired: 1 in]
  n182 = Bundle("spreadsheet string"=w4, "spreadsheet string"=w3, "spreadsheet string"=w2) -> (→"Settings Cluster":T48)  [unwired: 1 in]
